vi "CB Elevator Model.vi"(8 "dt":dbl=-1.0, 9 "G (gear ratio)":dbl, 10 "pulley radius (m)":dbl, 11 "mass (kg)":dbl) -> (3 "State Space Model":T2)   [LabVIEW 2020]
uses:
  Motors/CB Motor ID.ctl
  <vilib>/Analysis/Matrix/Datatypes/RealMatrix.ctl
  CB State Space.ctl
  <vilib>/Analysis/Matrix/NI_Matrix.lvlib
panel:
  out "D":T1
  out "C":T1
  out "A":T1
  out "B":T1
  in  "Motor ID":T3
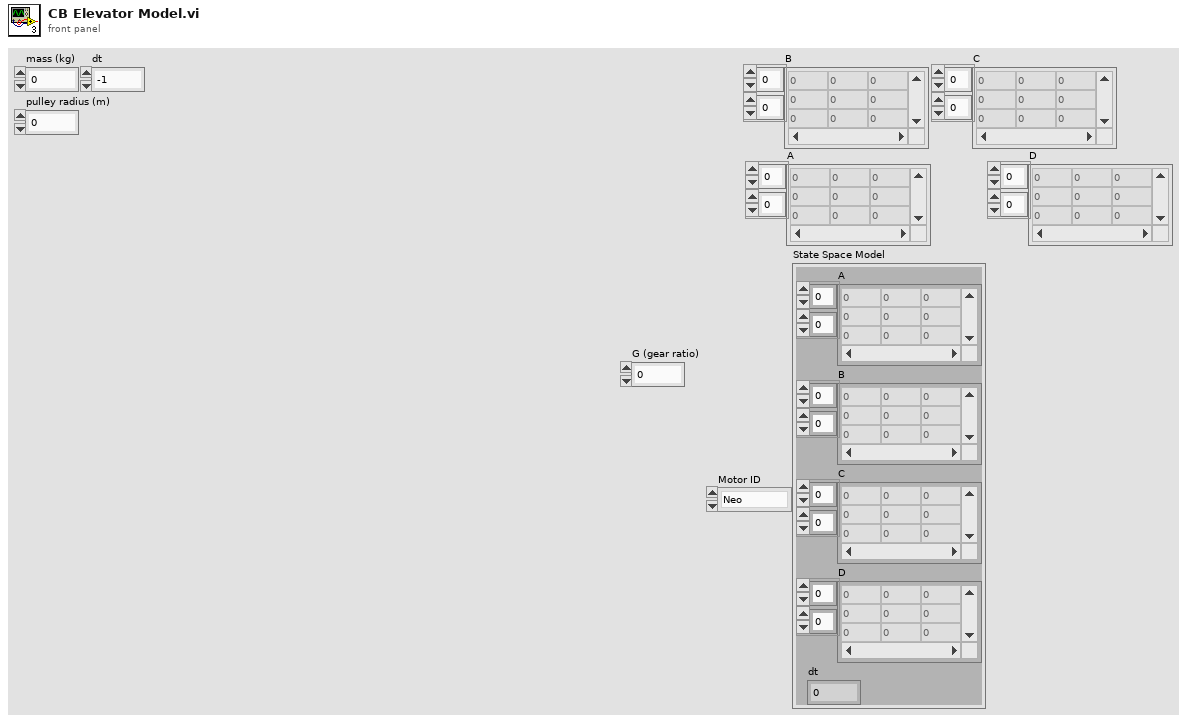
[diagram p1: front panel]
types:
  T1 = typedef "NI_Matrix.lvlib/RealMatrix.ctl" = dbl[][]
  T2 = typedef "CB State Space.ctl" = cluster{"A":T1, "B":T1, "C":T1, "D":T1, "dt":dbl}
  T3 = typedef "CB Motor ID.ctl" = enum16{"Neo", "Neo 550", "Falcon 500", "775pro"}
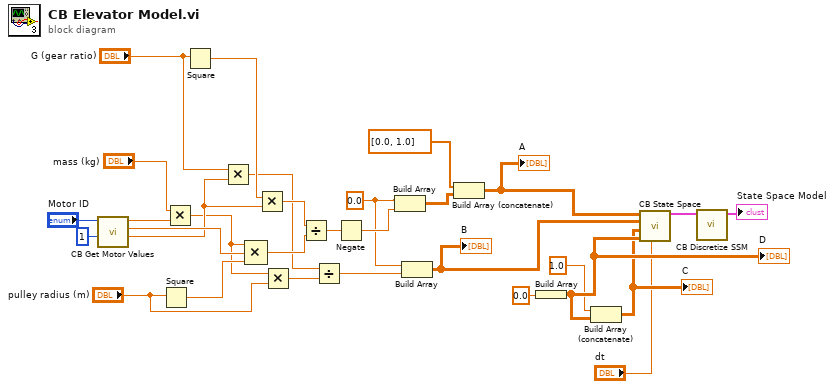
[diagram p0: block diagram]
diagram:
  w11 = 0.0
  n1 = call "CB Get Motor Values.vi"("num motors"=1, "Motor ID"="Motor ID") -> ("Kt"=w20:dbl, "Kv"=w26:dbl, "R"=w28:dbl)  [unwired: 6 in, 1 out]
  n2 = Square(x="pulley radius (m)") -> (x^2=w25:dbl)
  n3 = Multiply(x="mass (kg)", y=w28) -> (x*y=w18:dbl)
  n4 = Square(x="G (gear ratio)") -> (x^2=w24:dbl)
  n5 = Multiply(x="G (gear ratio)", y=w20) -> (x*y=w15:dbl)
  n6 = Compound Arithmetic op=MULTIPLY(w18, w26, w25) -> (w22:dbl)
  n7 = Multiply(x=w24, y=w20) -> (x*y=w23:dbl)
  n8 = Multiply(x=w18, y="pulley radius (m)") -> (x*y=w16:dbl)
  n9 = Divide(x=w23, y=w22) -> (x/y=w21:dbl)
  n10 = Divide(x=w15, y=w16) -> (x/y=w13:dbl)
  n11 = Negate(x=w21) -> (-x=w12:dbl)
  n12 = Build Array(w11, w12) -> (w10:T1)
  n13 = Build Array(w11, w13) -> (w8:T1)
  "B" <- w8
  n14 = Build Array (concatenate)(dbl[] [0.0, 1.0] ("element"), w10) -> (w9:T1)
  "A" <- w9
  n15 = Build Array(0.0) -> (w6:T1)
  "D" <- w6
  n16 = Build Array (concatenate)(1.0, w6) -> (w4:T1)
  "C" <- w4
  n17 = call "CB State Space.vi"("dt"="dt", "D"=w6, "C"=w4, "B"=w8, "A"=w9) -> ("State Space Model"=w2:T2)  [unwired: 5 in, 1 out]
  n18 = call "CB Discretize SSM.vi"("Cont SSM"=w2) -> ("State Space Model"=→"State Space Model":T2)  [unwired: 10 in]
